vi "Read Attributes.vi"(11 "Executioner in":refnum<class "Executioner.lvclass">) -> (3 "Executioner out":refnum<class "Executioner.lvclass">, 4 "Values":variant[](array[variant]), 6 "Names":string[](array[string]))   [LabVIEW 2017, in "Test Executive.lvlib" / "Executioner.lvclass"]
uses:
  <vilib>/gpm_packages/@cs/test-executive/Source/Test Executive/Executioner/Executioner.lvclass
  <vilib>/gpm_packages/@cs/test-executive/Source/Test Executive/Executioner/Executioner.lvclass/Executioner.ctl
  <vilib>/gpm_packages/@cs/lookup-table/Source/LookupTable/LookupTable.lvclass/LookupTable.ctl
  8c4f2e25-2f4b-4af1-8f35-350c449442ab.vi
  <vilib>/gpm_packages/@cs/lookup-table/Source/LookupTable/Read Table Reference.vi
  <vilib>/gpm_packages/@cs/lookup-table/Source/LookupTable/LookupTable.lvclass
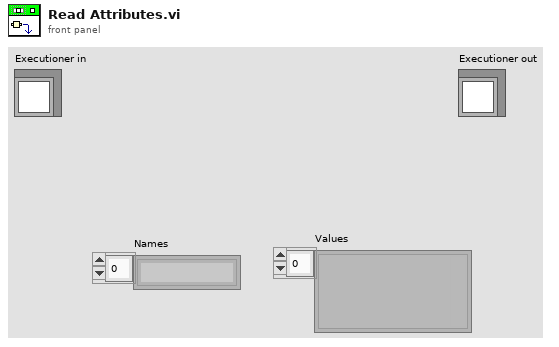
[diagram p1: front panel]
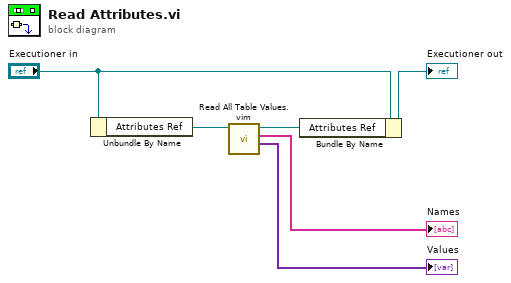
[diagram p0: block diagram]
diagram:
  n1 = Unbundle By Name("Executioner in") -> ("Attributes Ref"=w6:refnum<data-value>)
  n2 = call "Read All Table Values.vim"("LookupTable Reference"=w6) -> ("Values"=→"Values":variant[], "Names"=→"Names":string[], "LookupTable Reference Out"=w3:refnum<data-value>)  [unwired: 7 in, 1 out]
  n3 = Bundle By Name(cluster="Executioner in", "Attributes Ref"=w3) -> (→"Executioner out":refnum<class "Executioner.lvclass">)
